vi "SOM Host.vi"() -> ()   [LabVIEW 2014]
uses:
  <vilib>/rvi/interface/nirviOpenFPGA/nirviOpenFPGA.xnode
  <vilib>/rvi/interface/nirviMethod/nirviMethod.xnode
  <vilib>/FPGAPlugInAG/Dynamic/niLvFpga_Run_Dynamic.vi
  <vilib>/rvi/errors/niLvFpgaMergeErrorWithErrorCode.vi
  <vilib>/FPGAPlugInAG/Dynamic/niLvFpga_ReadFifo_Dynamic.vi
  <vilib>/rvi/interface/nirviCloseFPGA/nirviCloseFPGA.xnode
  <vilib>/FPGAPlugInAG/Dynamic/niLvFpga_StartFifo_Dynamic.vi
  <vilib>/FPGAPlugInAG/Dynamic/niLvFpga_Close_Dynamic.vi
  FPGA Bitfiles/DigilentPmodMIC-_FPGATarget_SPIFPGA_MxWWx5lIq+4.lvbitx
  SPI FPGA.vi
  <vilib>/FPGAPlugInAG/sbRIO-9651/niLvFpga_Open_sbRIO-9651.vi
  <vilib>/rvi/interface/common/dynamic/niFpgaDynamicAddResources.vi
panel:
  out "RT Loop Iterations":i32
  out "Waveform Chart":u64(graph)
  in  "stop":bool
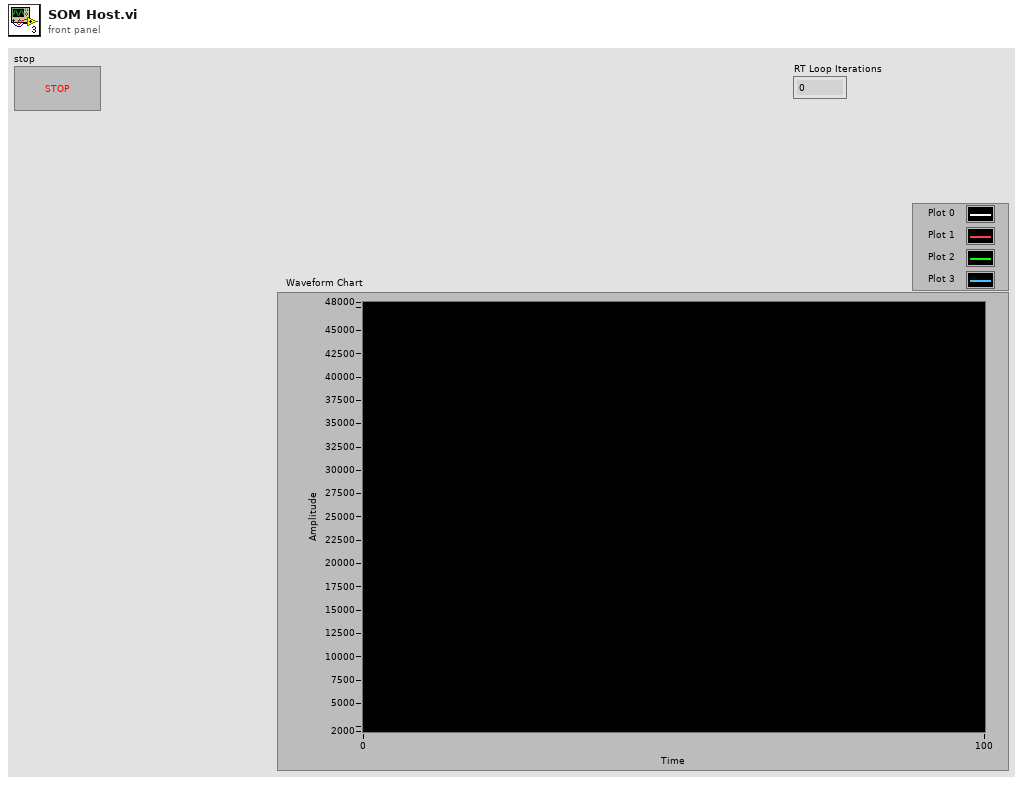
[diagram p1: front panel]
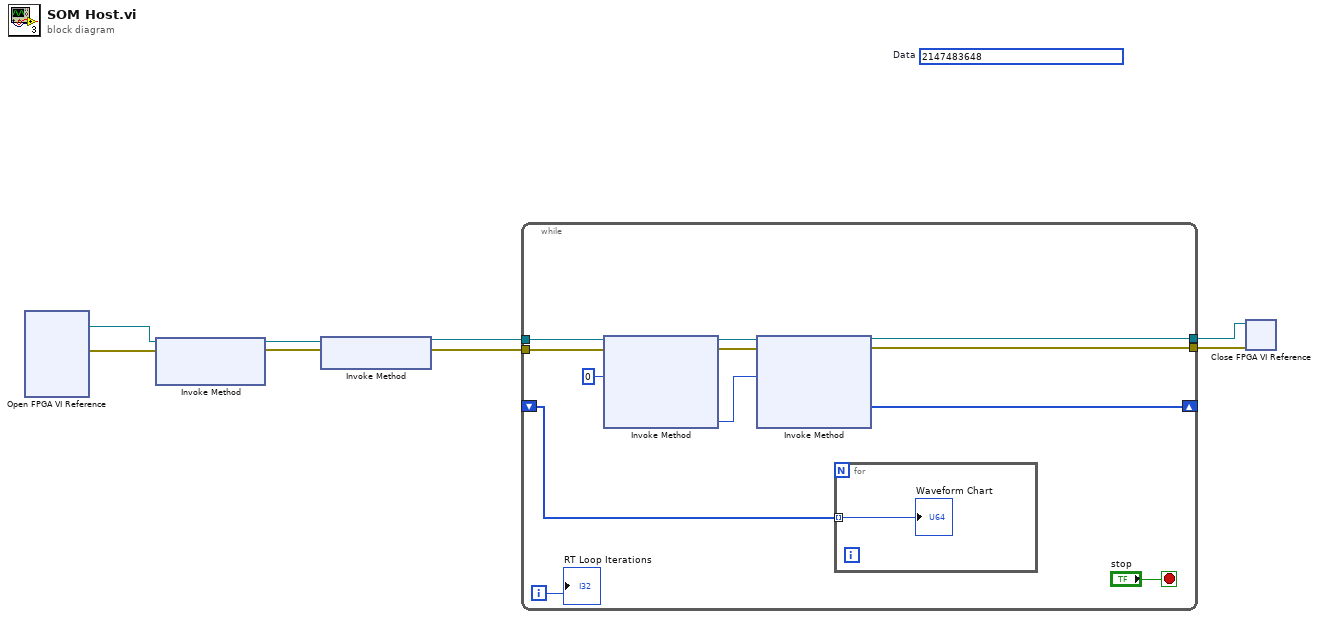
[diagram p0: block diagram]
diagram:
  (unwired) u64 2147483648  # Data
  n1 = xnode "Open FPGA VI Reference"() -> ("FPGA VI Reference Out"=w7:refnum<k20>, "error out"=w8:errorcluster)  [unwired: 2 in]
  n2 = xnode "Invoke Method"("FPGA VI Reference In"=w7, "error in"=w8) -> ("FPGA VI Reference Out"=w5:refnum<k20>, "error out"=w6:errorcluster)  [unwired: 1 in]
  n3 = xnode "Invoke Method"("FPGA VI Reference In"=w5, "error in"=w6) -> ("FPGA VI Reference Out"=w3:refnum<k20>, "error out"=w4:errorcluster)
  n4 = while {
    tunnel: w4 -> [w20]
    tunnel: w3 -> [w19]
    tunnel: [w10] -> w2
    tunnel: [w9] -> w1
    shift-right: [w13] -> _
    shift-left: _ -> [w11]
    i -> [w12]
    stop <- "stop" stop-if-true
    n5 = xnode "Invoke Method"("FPGA VI Reference In"=w19, "error in"=w20, "Number of Elements"=u32 0) -> ("FPGA VI Reference Out"=w17:refnum<k20>, "error out"=w16:errorcluster, "Elements Remaining"=w15:u32)  [unwired: 1 in, 1 out]
    n6 = xnode "Invoke Method"("FPGA VI Reference In"=w17, "error in"=w16, "Number of Elements"=w15) -> ("FPGA VI Reference Out"=w9:refnum<k20>, "error out"=w10:errorcluster, "Data"=w13:u64[])  [unwired: 1 in, 1 out]
    n7 = for {
      tunnel: w11 -> [w21] mode=indexing
      "Waveform Chart" <- w21
    }
    "RT Loop Iterations" <- w12
  }
  n8 = xnode "Close FPGA VI Reference"("FPGA VI Reference In"=w1, "error in"=w2) -> ()  [unwired: 1 out]
